vi "SoftwarePhase.vi"() -> ()   [LabVIEW 2012]
uses:
  <vilib>/imath/engines/lvmath/Plug In/_Char/NIMS_CH_character datatype.ctl
  <vilib>/Utility/inputDevices.llb/closeKeyboard.vi
  <vilib>/imath/engines/lvmath2/RunTimeEngine/ErrorHandling/NIMS_Finalize Error.vi
  <vilib>/imath/engines/lvmath2/RunTimeEngine/Managers/WorkSpace/UID Generator.vi
  <vilib>/imath/engines/lvmath2/RunTimeEngine/Managers/SymbolTable/Clear UID.vi
  <vilib>/imath/engines/lvmath/Plug In/_Char/NIMS_CH_Character RV to String.vi
  <vilib>/imath/engines/lvmath2/RunTimeEngine/NodeEndStatement/NIMS_NodeEndStatement_Output.vi
  <instcachedir>/0/NIMS_NodeEndStatement_Output_53EC0D466D134D7ABD903AC30B43404B.lvgen/NIMS_NodeEndStatement_Output_53EC0D466D134D7ABD903AC30B43404B_009.vi
  <vilib>/imath/engines/lvmath2/RunTimeEngine/RunTimeType/NIMS_RunTimeType_From StrictType (excl LVString).vi
  <instcachedir>/0/NIMS_RunTimeType_From StrictType (excl LVString)_AC52D965D0864706932D20A05968E122.lvgen/NIMS_RunTimeType_From StrictType (excl LVString)_AC52D965D0864706932D20A05968E122_001.vi
  <vilib>/imath/engines/lvmath2/RunTimeEngine/LocalVariableDefStatement/MC_LocalVariableDefStatement_Display.vi
  <vilib>/Utility/inputDevices.llb/keyboardAcquire.vi
  <vilib>/imath/engines/lvmath2/RunTimeEngine/Managers/SymbolTable/NIMS_WorkSpace.lvlib
panel:
  in  "Tab Control":T1(tab)
  out "Bump Sensor 2":bool
  out "Distance 2, CM":dbl
  out "IR Volts 2":dbl
  out "Red":dbl(knob) scale=0.0..100.0
  out "Green":dbl(knob) scale=0.0..100.0
  out "Blue":dbl(knob) scale=0.0..100.0
  out "Color Chosen":u32(colorbox)
  out "Bump Sensor 1":bool
  out "IR Volts 1":dbl
  out "Distance 1, CM":dbl
  in  "stop":bool
  out "Left Rudder":i32
  out "Right Rudder":i32
  in  "Rudders":i32(slide)=1500 scale=500.0..2500.0
  out "Port\nMotor":i32
  out "Starboard\nMotor":i32
  out "Port Speed":i32(knob) scale=1150.0..1750.0
  out "Starboard Speed":i32(knob) scale=1150.0..1750.0
  in  "Pan Camera":i32(slide)=1500 scale=500.0..2500.0
  out "Speed Balance":i32(knob) scale=-600.0..600.0
  in  "Step Size":i32=5
  in  "PC Status":i32=1
  out "String Received":string
  out "return count":u32
  out "bytes written":u32
  out "Blinky":bool
  in  "String":string="$CS1500P1500R1500L1500P1500H   1\n"
  in  "FULLSTOP":bool
  in  "VISA resource name":refnum<visa-resource-name>="COM7"
  # "ROBOT CONTROL VI\nSoftware Phase for Autonomy\n\nVPreston\n3/4/2014"
  # "Use this tab to make sure your sensors are happy and working properly."
  # "Motor Control"
  # "Direction of thrust"
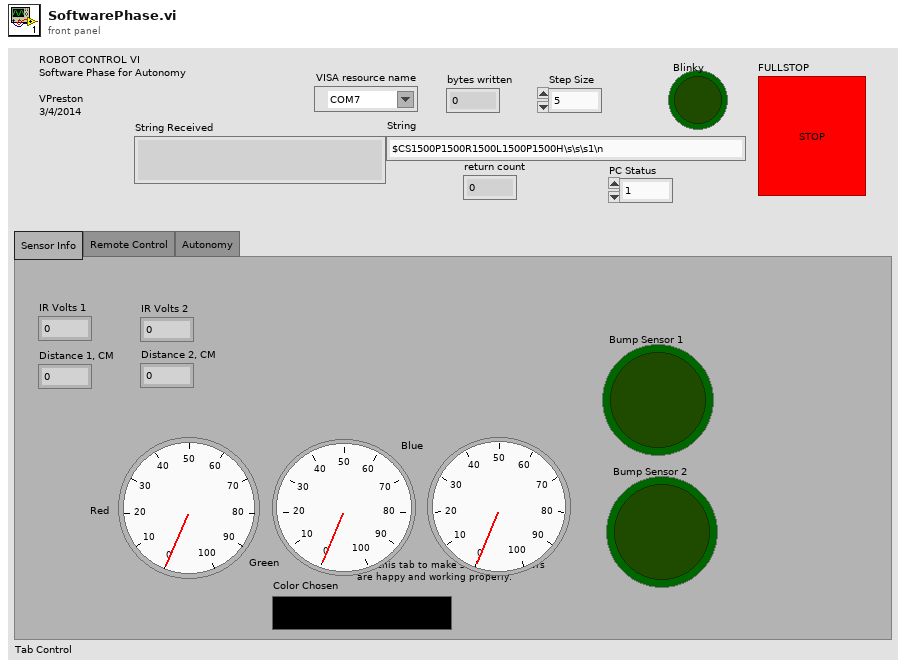
[diagram p1: front panel]
types:
  T1 = enum32{"Sensor Info", "Remote Control", "Autonomy"}
  T2 = enum16{"0", "1", "2", "3", "4", "5", "6", "7", "8", "9", "A", "B", "C", "D", "E", "F", "G", "H", "I", "J", "K", "L", "M", "N", "O", "P", "Q", "R", "S", "T", "U", "V", "W", "X", "Y", "Z", "F1", "F2", "F3", "F4", "F5", "F6", "F7", "F8", "F9", "F10", "F11", "F12", "F13", "F14", "F15", "ADD", "BACK", "BACKSLASH", "CAPITAL", "COMMA", "DECIMAL", "DELETE", "DIVIDE", "DOWN", "END", "EQUALS", "ESCAPE", "GRAVE (`)", "HOME", "INSERT", "LBRACKET", "LCONTROL", "LEFT", "L ALT", "LSHIFT", "LWIN", "MINUS", "MULTIPLY", "NEXT", "NUMLOCK", "NUMPAD_0", "NUMPAD_1", "NUMPAD_2", "NUMPAD_3", "NUMPAD_4", "NUMPAD_5", "NUMPAD_6", "NUMPAD_7", "NUMPAD_8", "NUMPAD_9", "PAUSE", "PERIOD", "PRIOR (PG UP)", "RBRACKET", "RCONTROL", "RETURN", "RIGHT", "R ALT", "RSHIFT", "RWIN", "SCROLL", "SEMICOLON", "SLASH", "SPACE", "SUBTRACT", "TAB", "UP", "ENTER (num pad)", "' (quote)"}[]
  T3 = enum16{"0", "1", "2", "3", "4", "5", "6", "7", "8", "9", "A", "B", "C", "D", "E", "F", "G", "H", "I", "J", "K", "L", "M", "N", "O", "P", "Q", "R", "S", "T", "U", "V", "W", "X", "Y", "Z", "F1", "F2", "F3", "F4", "F5", "F6", "F7", "F8", "F9", "F10", "F11", "F12", "F13", "F14", "F15", "ADD", "BACK", "BACKSLASH", "CAPITAL", "COMMA", "DECIMAL", "DELETE", "DIVIDE", "DOWN", "END", "EQUALS", "ESCAPE", "GRAVE (`)", "HOME", "INSERT", "LBRACKET", "LCONTROL", "LEFT", "L ALT", "LSHIFT", "LWIN", "MINUS", "MULTIPLY", "NEXT", "NUMLOCK", "NUMPAD_0", "NUMPAD_1", "NUMPAD_2", "NUMPAD_3", "NUMPAD_4", "NUMPAD_5", "NUMPAD_6", "NUMPAD_7", "NUMPAD_8", "NUMPAD_9", "PAUSE", "PERIOD", "PRIOR (PG UP)", "RBRACKET", "RCONTROL", "RETURN", "RIGHT", "R ALT", "RSHIFT", "RWIN", "SCROLL", "SEMICOLON", "SLASH", "SPACE", "SUBTRACT", "TAB", "UP", "ENTER (num pad)", "' (quote)"}
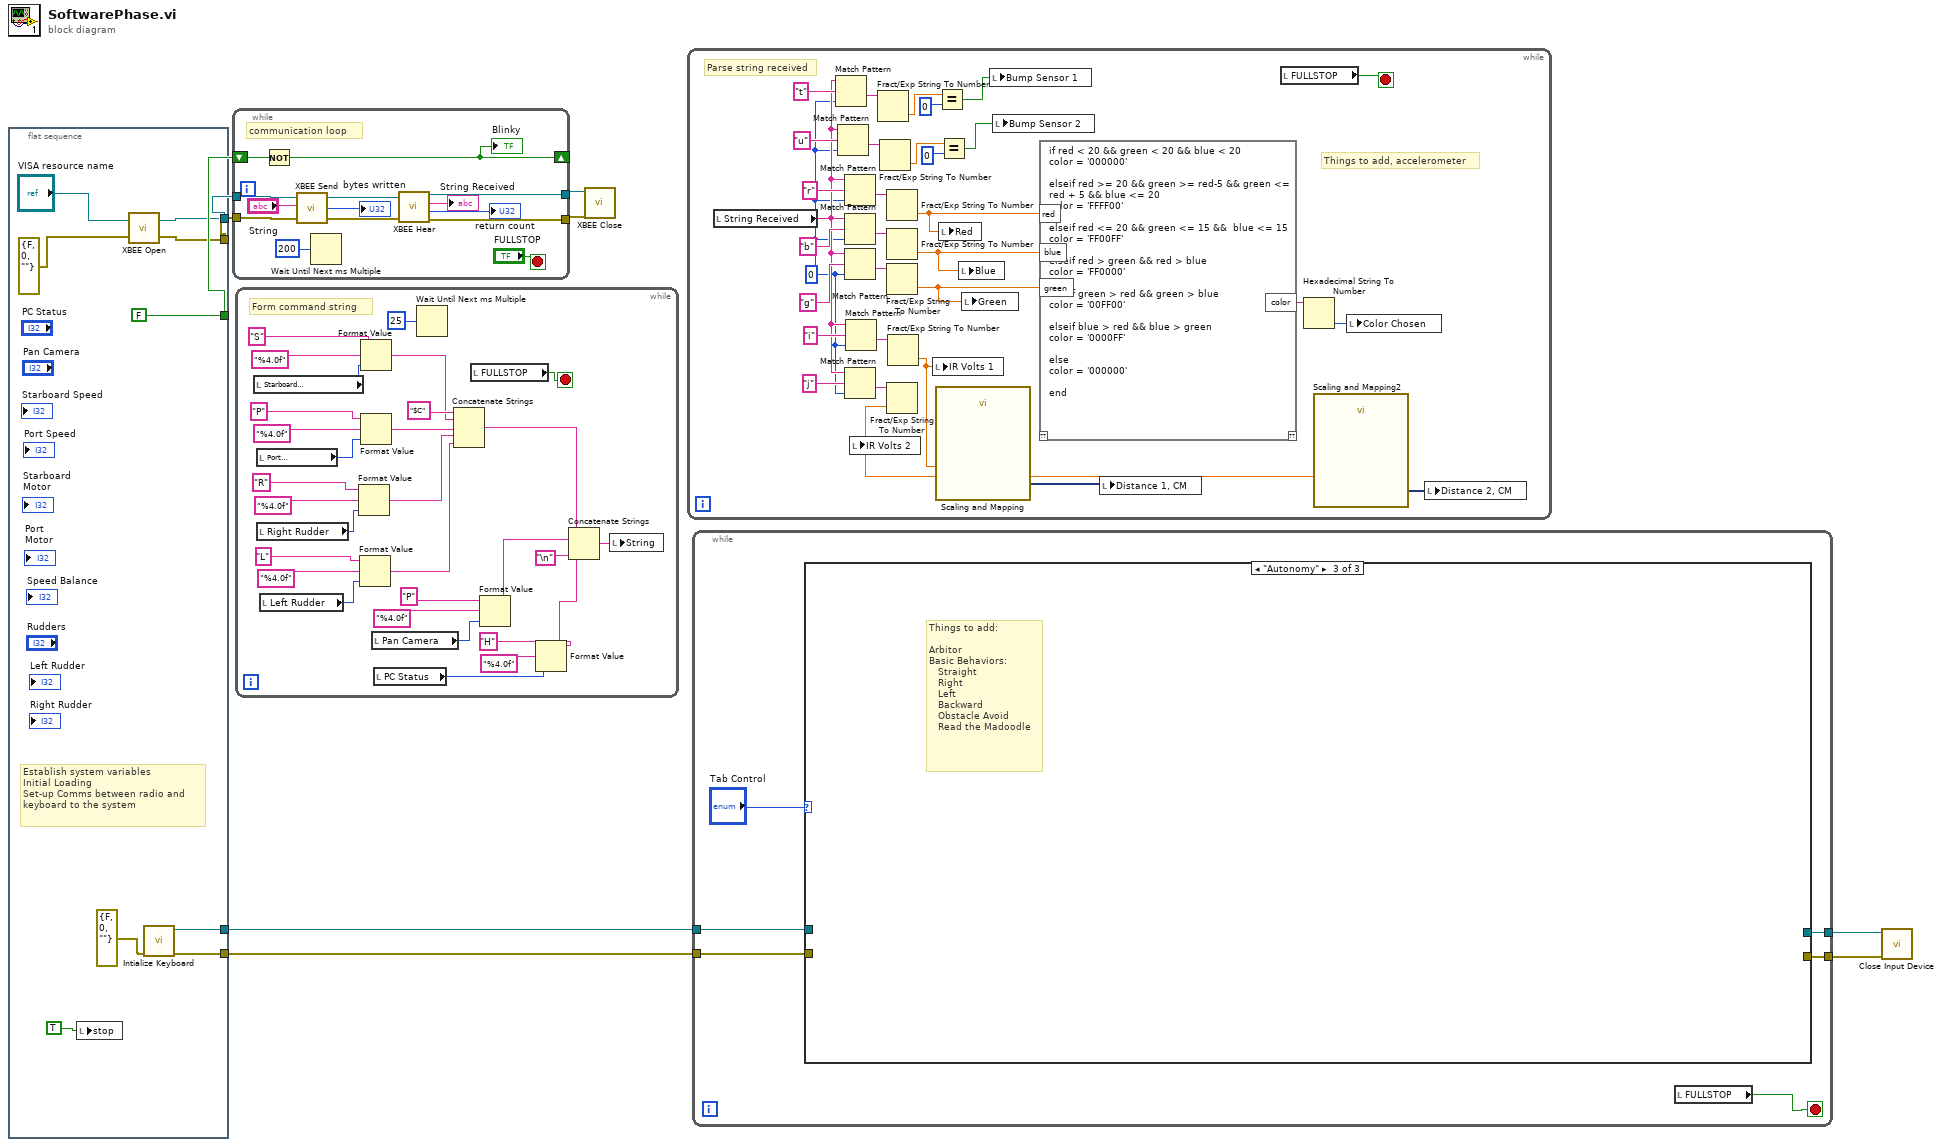
[diagram p0: block diagram]
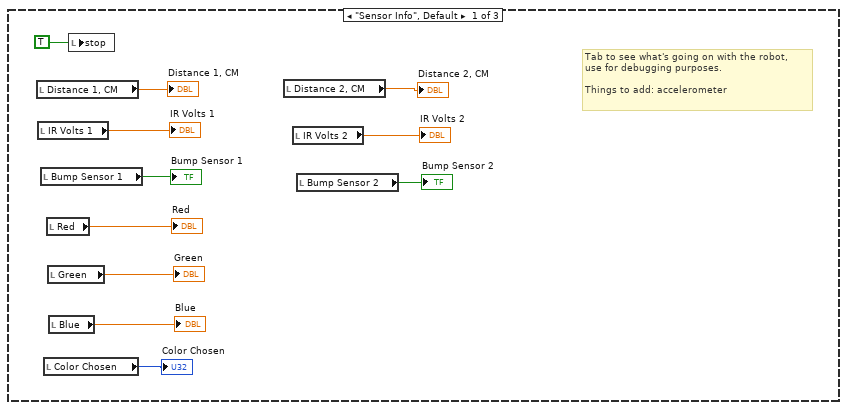
[diagram p2: hidden frame]
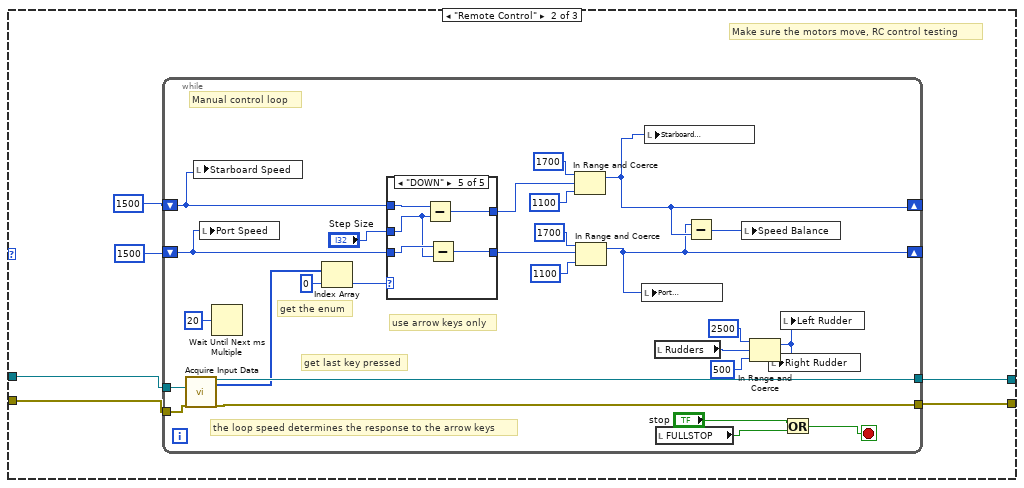
[diagram p3: hidden frame]
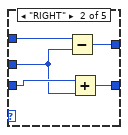
[diagram p5: hidden frame]
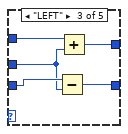
[diagram p6: hidden frame]
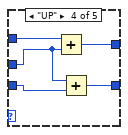
[diagram p7: hidden frame]
diagram:
  n1 = flat-sequence {
    tunnel: [w18] -> w9
    tunnel: [w17] -> w8
    tunnel: [FALSE] -> w5
    tunnel: [w12] -> w4
    tunnel: [w11] -> w3
    frame #0 {
      # "Establish system variables\nInitial Loading\nSet-up Comms between radio and\nkeyboard to the system"
      n2 = local write "stop"(TRUE) -> ()
      n3 = call "XBEE Open.vi"("error in"=errorcluster {"status"=FALSE, "code"=0, "source"=""}, "VISA resource name"="VISA resource name") -> ("error out"=w17:errorcluster, "VISA resource name out"=w18:refnum<visa-resource-name>)
      n4 = call <vilib>:"Intialize Keyboard.vi"("error in (no error)"=errorcluster {"status"=FALSE, "code"=0, "source"=""}) -> ("error out"=w11:errorcluster, "device ID"=w12:refnum<k1>)  [unwired: 9 in]
    }
  }
  n5 = while {
    tunnel: w9 -> [w31]
    tunnel: w8 -> [w30]
    tunnel: [w25] -> w7
    tunnel: [w24] -> w6
    shift-right: [w28] -> _
    shift-left: w5 -> [w29]
    stop <- "FULLSTOP" stop-if-true
    # "communication loop"
    n6 = Not(x=w29) -> (.not. x?=w28:bool)
    "Blinky" <- w28
    n7 = call "XBEE Send.vi"("error in (no error)"=w30, "String"="String", "VISA resource name"=w31) -> ("error out"=w21:errorcluster, "return count"=→"bytes written":u32, "VISA resource name out"=w22:refnum<visa-resource-name>)
    n8 = Wait Until Next ms Multiple(millisecond multiple=u32 200) -> ()  [unwired: 1 out]
    n9 = call "XBEE Hear.vi"("VISA resource name"=w22, "error in (no error)"=w21) -> ("VISA resource name out"=w25:refnum<visa-resource-name>, "String Received"=→"String Received":string, "return count"=→"return count":u32, "error out"=w24:errorcluster)
  }
  n10 = while {
    stop <- w62 stop-if-true
    # "Form command string"
    n11 = local read "Starboard\nMotor"() -> (w59:i32)
    n12 = local read "Port\nMotor"() -> (w56:i32)
    n13 = local read "Right Rudder"() -> (w50:i32)
    n14 = local read "Left Rudder"() -> (w47:i32)
    n15 = Format Value(string ("")="R", format string="%4.0f", value (0)=w50) -> (output string=w46:string)
    n16 = Format Value(string ("")="L", format string="%4.0f", value (0)=w47) -> (output string=w45:string)
    n17 = Format Value(string ("")="S", format string="%4.0f", value (0)=w59) -> (output string=w54:string)
    n18 = Format Value(string ("")="P", format string="%4.0f", value (0)=w56) -> (output string=w53:string)
    n19 = local read "Pan Camera"() -> (w41:i32)
    n20 = local read "PC Status"() -> (w38:i32)
    n21 = Wait Until Next ms Multiple(millisecond multiple=u32 25) -> ()  [unwired: 1 out]
    n22 = Concatenate Strings("$C", w54, w53, w46, w45) -> (w37:string)
    n23 = local read "FULLSTOP"() -> (w62:bool)
    n24 = Format Value(string ("")="P", format string="%4.0f", value (0)=w41) -> (output string=w36:string)
    n25 = Format Value(string ("")="H", format string="%4.0f", value (0)=w38) -> (output string=w35:string)
    n26 = Concatenate Strings(w37, w36, w35, "\n") -> (w42:string)
    n27 = local write "String"(w42) -> ()
  }
  n28 = call "XBEE Close.vi"("error in (no error)"=w6, "VISA resource name"=w7) -> ()
  n29 = while {
    stop <- w94 stop-if-true
    w64 = 0 ("offset (0)")
    # "Things to add, accelerometer"
    # "Parse string received"
    n30 = local read "String Received"() -> (w65:string)
    n31 = Match Pattern(string=w65, regular expression="t", offset (0)=w64) -> (after substring=w81:string)  [unwired: 3 out]
    n32 = Match Pattern(string=w65, regular expression="u", offset (0)=w64) -> (after substring=w66:string)  [unwired: 3 out]
    n33 = Match Pattern(string=w65, regular expression="r", offset (0)=w64) -> (after substring=w84:string)  [unwired: 3 out]
    n34 = Match Pattern(string=w65, regular expression="b", offset (0)=w64) -> (after substring=w82:string)  [unwired: 3 out]
    n35 = Match Pattern(string=w65, regular expression="g", offset (0)=w64) -> (after substring=w83:string)  [unwired: 3 out]
    n36 = Match Pattern(string=w65, regular expression="j", offset (0)=w64) -> (after substring=w72:string)  [unwired: 3 out]
    n37 = Match Pattern(string=w65, regular expression="i", offset (0)=w64) -> (after substring=w85:string)  [unwired: 3 out]
    n38 = Fract/Exp String To Number(string=w81) -> (number=w92:dbl)  [unwired: 3 in, 1 out]
    n39 = Fract/Exp String To Number(string=w66) -> (number=w69:dbl)  [unwired: 3 in, 1 out]
    n40 = Fract/Exp String To Number(string=w84) -> (number=w78:dbl)  [unwired: 3 in, 1 out]
    n41 = Fract/Exp String To Number(string=w82) -> (number=w77:dbl)  [unwired: 3 in, 1 out]
    n42 = Fract/Exp String To Number(string=w83) -> (number=w76:dbl)  [unwired: 3 in, 1 out]
    n43 = Fract/Exp String To Number(string=w72) -> (number=w71:dbl)  [unwired: 3 in, 1 out]
    n44 = local write "IR Volts 2"(w71) -> ()
    n45 = Fract/Exp String To Number(string=w85) -> (number=w75:dbl)  [unwired: 3 in, 1 out]
    n46 = local write "IR Volts 1"(w75) -> ()
    n47 = call "Scaling and Mapping"("Signals"=w75) -> ("Scaled Signals"=w74:dynamicdata)  [unwired: 9 in, 1 out]
    n48 = Equal?(x=w92, y=0) -> (x = y?=w79:bool)
    n49 = Equal?(x=w69, y=0) -> (x = y?=w63:bool)
    n50 = local write "Red"(w78) -> ()
    n51 = local write "Blue"(w77) -> ()
    n52 = local write "Green"(w76) -> ()
    n53 = local write "Bump Sensor 1"(w79) -> ()
    n54 = local write "Bump Sensor 2"(w63) -> ()
    n55 = mathscript code="if red < 20 && green < 20 && blue < 20\ncolor = '000000'\n\nelseif red >= 20 && green >= red-5 && green <= red + 5 && blue <= 20\ncolor = 'FFFF00'\n\nelseif red <= 20 && green <= 15 &&  blue <= 15\ncolor = 'FF00FF'\n\nelseif red > green && red > blue\ncolor = 'FF0000'\n\nelseif green > red && green > blue\ncolor = '00FF00'\n\nelseif blue > red && blue > green\ncolor = '0000FF' \n\nelse\ncolor = '000000'\n\nend"("red"=w78, "blue"=w77, "green"=w76) -> ("color"=w93:string)  [unwired: 1 in, 1 out]
    n56 = local write "Distance 1, CM"(w74) -> ()
    n57 = local read "FULLSTOP"() -> (w94:bool)
    n58 = Hexadecimal String To Number(string=w93) -> (number=w80:u32)  [unwired: 2 in, 1 out]
    n59 = call "Scaling and Mapping2"("Signals"=w71) -> ("Scaled Signals"=w70:dynamicdata)  [unwired: 9 in, 1 out]
    n60 = local write "Color Chosen"(w80) -> ()
    n61 = local write "Distance 2, CM"(w70) -> ()
  }
  n62 = while {
    tunnel: w4 -> [w384]
    tunnel: w3 -> [w383]
    tunnel: [w382] -> w2
    tunnel: [w381] -> w1
    stop <- w385 stop-if-true
    n63 = case shown="\"Autonomy\"" "Tab Control" {
      tunnel: w384 -> [_ w403 _]
      tunnel: w383 -> [_ w402 _]
      tunnel: [_ w399 _] -> w382
      tunnel: [_ w398 _] -> w381
      frame "Sensor Info", Default {
        # "Tab to see what's going on with the robot, \nuse for debugging purposes.  \n\nThings to add: accelerometer"
        n64 = local read "Distance 1, CM"() -> (→"Distance 1, CM":dbl)
        n65 = local read "IR Volts 1"() -> (→"IR Volts 1":dbl)
        n66 = local read "Bump Sensor 1"() -> (→"Bump Sensor 1":bool)
        n67 = local read "Color Chosen"() -> (→"Color Chosen":u32)
        n68 = local read "Red"() -> (→"Red":dbl)
        n69 = local read "Green"() -> (→"Green":dbl)
        n70 = local read "Blue"() -> (→"Blue":dbl)
        n71 = local write "stop"(TRUE) -> ()
        n72 = local read "Distance 2, CM"() -> (→"Distance 2, CM":dbl)
        n73 = local read "IR Volts 2"() -> (→"IR Volts 2":dbl)
        n74 = local read "Bump Sensor 2"() -> (→"Bump Sensor 2":bool)
      }
      frame "Remote Control" {
        # "Make sure the motors move, RC control testing"
        n75 = while {
          tunnel: [w430] -> w398
          tunnel: [w429] -> w399
          shift-right: [w413] -> _
          shift-left: 1500 -> [w415]
          shift-right: [w412] -> _
          shift-left: 1500 -> [w414]
          tunnel: w403 -> [w405]
          tunnel: w402 -> [w404]
          stop <- w406 stop-if-true
          # "use arrow keys only"
          # "Manual control loop"
          # "get the enum"
          # "the loop speed determines the response to the arrow keys"
          # "get last key pressed"
          n76 = call-poly <vilib>:"Acquire Input Data.vi"("device ID"=w405, "error in (no error)"=w404) -> ("device ID"=w429:refnum<k1>, "keys pressed"=w428:T2, "error out"=w430:errorcluster)  [unwired: 15 in]
          n77 = local write "Starboard Speed"(w415) -> ()
          n78 = local write "Port Speed"(w414) -> ()
          n79 = Wait Until Next ms Multiple(millisecond multiple=u32 20) -> ()  [unwired: 1 out]
          n80 = Index Array(array=w428, index=0) -> (element=w426:T3)
          n81 = case shown="\"DOWN\"" w426 {
            tunnel: w415 -> [w432 w434 w439 w447 w452]
            tunnel: [w432 w435 w440 w446 w451] -> w424
            tunnel: w414 -> [w431 w437 w441 w444 w450]
            tunnel: [w431 w436 w442 w443 w448] -> w416
            tunnel: "Step Size" -> [_ w433 w438 w445 w449]
            frame "0", Default {
            }
            frame "RIGHT" {
              n82 = Subtract(x=w434, y=w433) -> (x-y=w435:i32)
              n83 = Add(x=w437, y=w433) -> (x+y=w436:i32)
            }
            frame "LEFT" {
              n84 = Subtract(x=w441, y=w438) -> (x-y=w442:i32)
              n85 = Add(x=w439, y=w438) -> (x+y=w440:i32)
            }
            frame "UP" {
              n86 = Add(x=w447, y=w445) -> (x+y=w446:i32)
              n87 = Add(x=w445, y=w444) -> (x+y=w443:i32)
            }
            frame "DOWN" {
              n88 = Subtract(x=w452, y=w449) -> (x-y=w451:i32)
              n89 = Subtract(x=w450, y=w449) -> (x-y=w448:i32)
            }
          }
          n90 = In Range and Coerce(upper limit=1700, x=w424, lower limit=1100) -> (coerced(x)=w413:i32)  [unwired: 1 out]
          n91 = In Range and Coerce(upper limit=1700, x=w416, lower limit=1100) -> (coerced(x)=w412:i32)  [unwired: 1 out]
          n92 = local write "Port\nMotor"(w412) -> ()
          n93 = local write "Starboard\nMotor"(w413) -> ()
          n94 = local read "Rudders"() -> (w410:i32)
          n95 = local read "FULLSTOP"() -> (w407:bool)
          n96 = Subtract(x=w412, y=w413) -> (x-y=w411:i32)
          n97 = local write "Speed Balance"(w411) -> ()
          n98 = In Range and Coerce(upper limit=2500, x=w410, lower limit=500) -> (coerced(x)=w409:i32)  [unwired: 1 out]
          n99 = local write "Right Rudder"(w409) -> ()
          n100 = local write "Left Rudder"(w409) -> ()
          n101 = Or(x="stop", y=w407) -> (x .or. y?=w406:bool)
        }
      }
      frame "Autonomy" {
        # "Things to add: \n\nArbitor\nBasic Behaviors:\n   Straight\n   Right\n   Left\n   Backward\n   Obstacle Avoid\n   Read the Madoodle"
      }
    }
    n102 = local read "FULLSTOP"() -> (w385:bool)
  }
  n103 = call-poly <vilib>:"Close Input Device.vi"("error in (no error)"=w1, "device ID"=w2) -> ()  [unwired: 8 in, 1 out]
